vi "NI VeriStand - Asynchronous Disconnect from System.vi"(6 "Undeploy System Definition (F)":bool, 8 "error in (no error)":errorcluster, 10 "Password (\"\")":string, 11 "WorkspaceManager in":T1) -> (0 "error out":errorcluster, 3 "WorkspaceManager out":T1)   [LabVIEW 2020, in "NI_VS Workspace ExecutionAPI.lvlib"]
uses:
  <vilib>/NI VeriStand/Execution/Workspace/NI_VS Workspace ExecutionAPI.lvlib
  <vilib>/NI VeriStand/Execution/Workspace/WorkspaceAPI.ctl
  NationalInstruments.VeriStand.ClientAPI
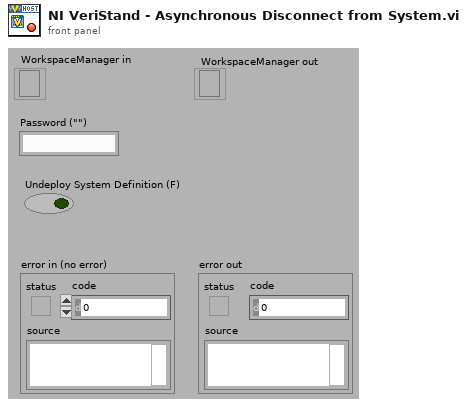
[diagram p1: front panel]
types:
  T1 = typedef "NI_VS Workspace ExecutionAPI.lvlib/WorkspaceAPI.ctl" = refnum<k24>
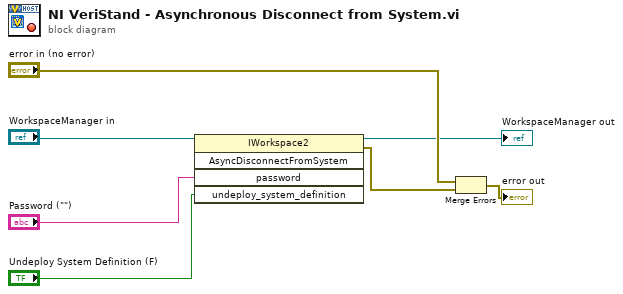
[diagram p0: block diagram]
diagram:
  n1 = invoke class="IWorkspace2" method="AsyncDisconnectFromSystem"(reference="WorkspaceManager in", "password"="Password (\"\")", "undeploy_system_definition"="Undeploy System Definition (F)") -> (reference out=→"WorkspaceManager out":T1, error out=w1:errorcluster)  [unwired: 2 in, 3 out]
  n2 = Merge Errors("error in (no error)", w1) -> (→"error out":errorcluster)
